vi "Calc Error.vi"(10 "YInput":dbl[](array[numeric]), 11 "Neuron Stucture In":T1) -> (3 "Neuron Stucture Out":T1)   [LabVIEW 2012]
uses:
  NeuronData.ctl
panel:
  # "Chuck Streb Dec2007"
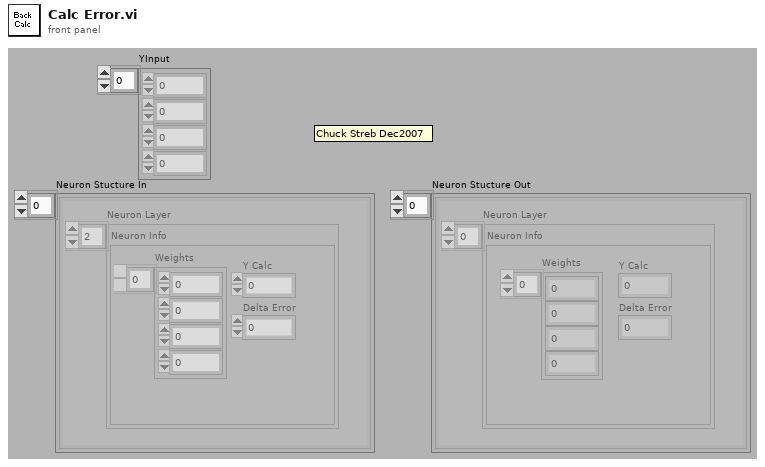
[diagram p1: front panel]
types:
  T1 = typedef "NeuronData.ctl" = cluster{"Neuron Layer":cluster{"Weights":dbl[], "Y Calc":dbl, "Delta Error":dbl}[]}[]
  T2 = cluster{"Weights":dbl[], "Y Calc":dbl, "Delta Error":dbl}[]
  T3 = cluster{"Weights":dbl[], "Y Calc":dbl, "Delta Error":dbl}
  T4 = cluster{"Neuron Layer":cluster{"Weights":dbl[], "Y Calc":dbl, "Delta Error":dbl}[]}
  T5 = cluster{"Neuron Layer":cluster{"Weights":dbl[], "Y Calc":dbl, "Delta Error":dbl}[]}[]
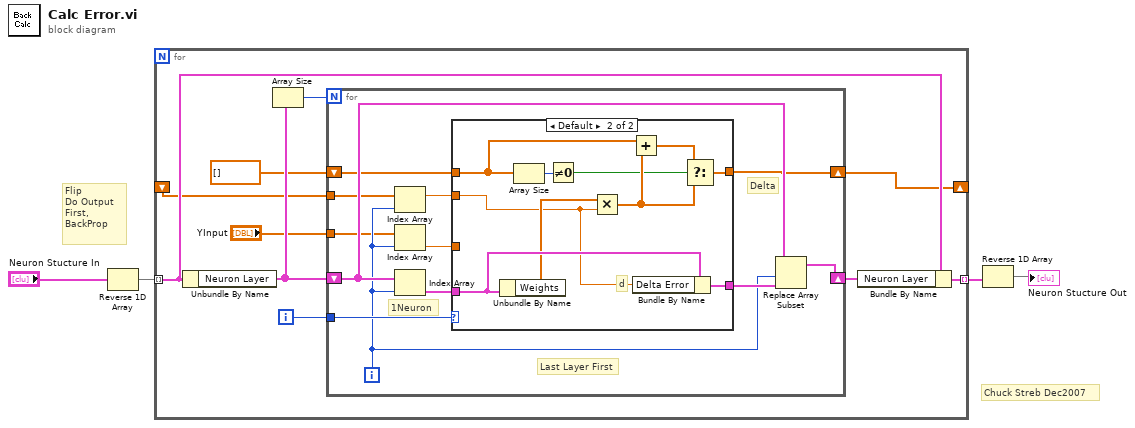
[diagram p0: block diagram]
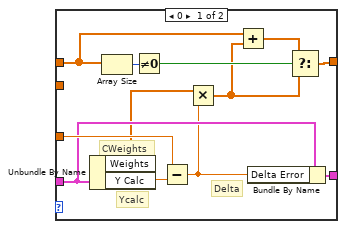
[diagram p2: hidden frame]
diagram:
  # "Chuck Streb Dec2007"
  # "Flip\nDo Output\nFirst,\nBackProp"
  n1 = Reverse 1D Array(array="Neuron Stucture In") -> (reversed array=w3:T1)
  n2 = for {
    tunnel: w3 -> [w12] mode=indexing
    tunnel: [w10] -> w2 mode=indexing
    shift-right: [w8] -> _
    shift-left: _ -> [w6]
    i -> [w9]
    n3 = Unbundle By Name(w12) -> ("Neuron Layer"=w13:T2)
    n4 = Array Size(array=w13) -> (size(s)=w14:i32)
    n5 = for {
      N: w14 -> [_]
      shift-right: [w23] -> w11
      shift-left: w13 -> [w22]
      tunnel: w9 -> [w26]
      shift-right: [w21] -> w8
      shift-left: dbl[] [] -> [w20]
      tunnel: w6 -> [w19]
      tunnel: "YInput" -> [w16]
      i -> [w17]
      # "Delta"
      # "1Neuron"
      # "Last Layer First"
      n6 = Index Array(array=w19, index=w17) -> (element=w18:dbl)
      n7 = Index Array(array=w16, index=w17) -> (element=w15:dbl)
      n8 = Index Array(array=w22, index=w17) -> (element=w25:T3)
      n9 = case shown="Default" w26 {
        tunnel: w25 -> [w37 w48]
        tunnel: w15 -> [w38 _]
        tunnel: [w36 w47] -> w24
        tunnel: [w28 w40] -> w21
        tunnel: w20 -> [w31 w45]
        tunnel: w18 -> [_ w39]
        frame 0 {
          # "Delta"
          # "CWeights"
          # "Ycalc"
          n10 = Unbundle By Name(w37) -> ("Weights"=w33:dbl[], "Y Calc"=w34:dbl)
          n11 = Array Size(array=w31) -> (size(s)=w32:i32)
          n12 = Not Equal To 0?(x=w32) -> (x != 0?=w30:bool)
          n13 = Subtract(x=w38, y=w34) -> (x-y=w35:dbl)
          n14 = Multiply(x=w33, y=w35) -> (x*y=w27:dbl[])
          n15 = Add(x=w31, y=w27) -> (x+y=w29:dbl[])
          n16 = Bundle By Name(cluster=w37, "Delta Error"=w35) -> (w36:T3)
          n17 = Select(t=w29, s=w30, f=w27) -> (s? t:f=w28:dbl[])
        }
        frame Default {
          # "d"
          n18 = Unbundle By Name(w48) -> ("Weights"=w46:dbl[])
          n19 = Array Size(array=w45) -> (size(s)=w44:i32)
          n20 = Not Equal To 0?(x=w44) -> (x != 0?=w41:bool)
          n21 = Multiply(x=w46, y=w39) -> (x*y=w42:dbl[])
          n22 = Add(x=w45, y=w42) -> (x+y=w43:dbl[])
          n23 = Bundle By Name(cluster=w48, "Delta Error"=w39) -> (w47:T3)
          n24 = Select(t=w43, s=w41, f=w42) -> (s? t:f=w40:dbl[])
        }
      }
      n25 = Replace Array Subset(array=w22, new element=w24, index=w17) -> (w23:T2)
    }
    n26 = Bundle By Name(cluster=w12, "Neuron Layer"=w11) -> (w10:T4)
  }
  n27 = Reverse 1D Array(array=w2) -> (reversed array=→"Neuron Stucture Out":T5)
